vi "读.vi"(8 "错误输入（无错误）":errorcluster, 9 "字数":string, 10 "开始字":string, 11 "VISA资源名称":refnum<visa-resource-name>) -> (0 "错误输出":errorcluster, 2 "读取缓冲区":string, 3 "VISA资源名称输出":refnum<visa-resource-name>)   [LabVIEW 2017]
panel:
  in  "命令码":string="RD"
  in  "节点号":string="00"
  # "通讯格式说明：\n   发送：\n     读：          起始符        节点号                 命令码        开始字             字数         FCS校验码   终止符\n                        @              00                       RD          0000              0002                \n起始符：必须以@开始\n节点号：默认是00，由DM6648和DM6653指定\n命令码：RD（DM数据区读）\n开始字：0000（个人理解是起始地址）（10进制数据）\n字数：0002（要读取的字的个数）（10进制数据）\nFCS校验码：\n终止符：*CR（由*和回车组成）（一定要组合，一次最多字符长度是131超过之后利用的是分隔符来读取的）\n\n\n\n\n\n     写：          起始符        节点号           命令码        开始字        第一个数据（字）  第二个数据（字）      FCS校验码    终止符\n                        @              00                WD          0000              0001                    0010\n起始符：必须以@开始\n节点号：默认是00，由DM6648和DM6653指定\n命令码：WD（DM数据区写）\n开始字：0000（个人理解是起始地址）（10进制数据）\n第一/二个数据（字）：0001/0010（写入的数据1和16）（16进制数据）\nFCS校验码：\n终止符：*CR（由*和回车组成）（一定要组合，一次最多字符长度是131超过之后利用的是分隔符来读取的）"
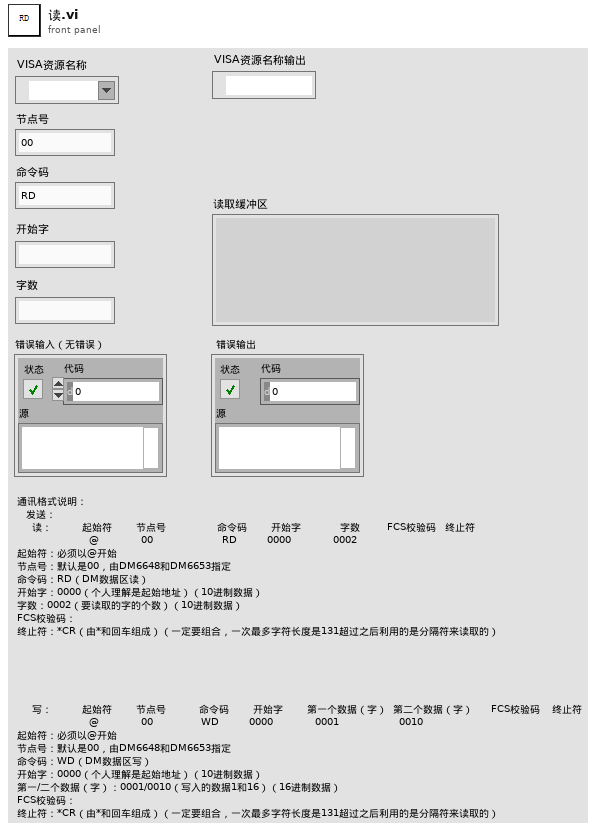
[diagram p1: front panel]
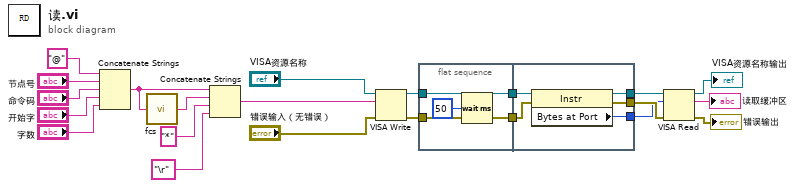
[diagram p0: block diagram]
diagram:
  n1 = Concatenate Strings("@", "节点号", "命令码", "开始字", "字数") -> (w18:string)
  n2 = call "fcs .vi"("string"=w18) -> ("frame check sum"=w17:string)
  n3 = Concatenate Strings(w18, w17, "*" ("搜索字符串"), "\r" ("搜索字符串")) -> (w15:string)
  n4 = VISA Write(VISA resource name="VISA资源名称", write buffer=w15, error in (no error)="错误输入（无错误）") -> (VISA resource name out=w7:refnum<visa-resource-name>, error out=w6:errorcluster)  [unwired: 1 out]
  n5 = flat-sequence {
    tunnel: [w24] -> w14
    tunnel: w7 -> [w24]
    tunnel: w6 -> [w23]
    tunnel: [w23] -> w13
    tunnel: w14 -> [w30]
    tunnel: w13 -> [w29]
    tunnel: [w28] -> w12
    tunnel: [w27] -> w11
    tunnel: [w26] -> w10
    frame #0 {
      n6 = Wait (ms)(milliseconds to wait=u32 50 ("等待时间（毫秒）")) -> ()  [unwired: 1 out]
    }
    frame #1 {
      n7 = property class="Instr"(reference=w30, error in=w29) -> (reference out=w28:refnum<visa-resource-name>, error out=w27:errorcluster, "Bytes at Port"=w26:u32)
    }
  }
  n8 = VISA Read(VISA resource name=w12, byte count=w10, error in (no error)=w11) -> (VISA resource name out=→"VISA资源名称输出":refnum<visa-resource-name>, read buffer=→"读取缓冲区":string, error out=→"错误输出":errorcluster)  [unwired: 1 out]
